vi "R ead.vi"(8 "error in (no error)":errorcluster, 10 "Start address":string, 11 "MelsecTCP in":refnum<class "MelsecMcNet.lvclass">) -> (0 "error out":errorcluster, 2 "Bools":bool, 3 "MelsecTCP out":refnum<class "MelsecMcNet.lvclass">)   [LabVIEW 2020]
uses:
  C:/Users/Fred Guo/Desktop/API_Salcomp_CMES/Libraries/HslCommunication/HslCommunication.dll
  HslCommunication.dll
  MelsecMcNet.lvclass
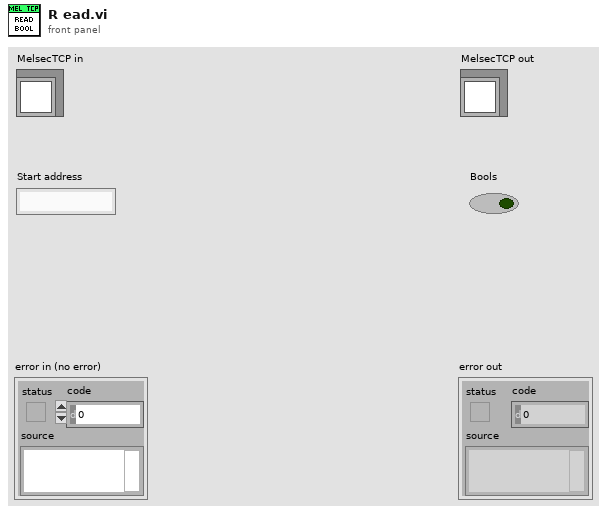
[diagram p1: front panel]
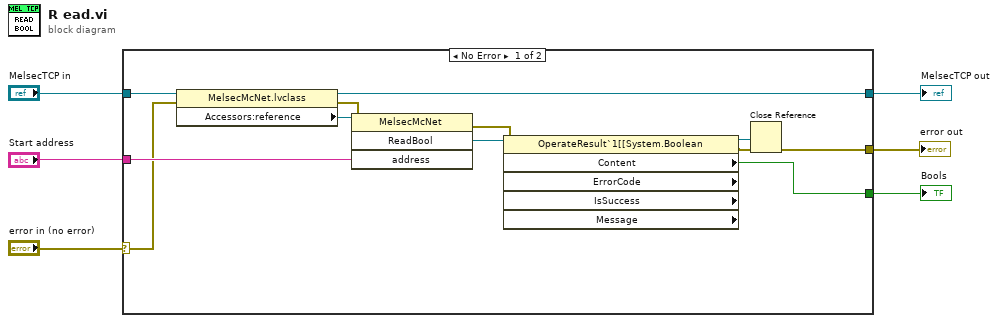
[diagram p0: block diagram]
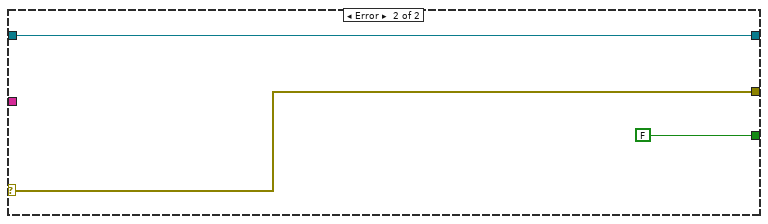
[diagram p2: hidden frame]
diagram:
  n1 = case shown="No Error" "error in (no error)" {
    selector: "error in (no error)" -> [w7 w21]
    tunnel: "MelsecTCP in" -> [w18 w19]
    tunnel: [w17 w19] -> w5
    tunnel: "Start address" -> [w15 _]
    tunnel: [w10 w21] -> w3
    tunnel: [w8 FALSE ("Content")] -> w2
    frame No Error {
      n2 = property class="MelsecMcNet.lvclass"(reference=w18, error in=w7) -> (reference out=w17:refnum<class "MelsecMcNet.lvclass">, error out=w13:errorcluster, "Accessors:reference"=w16:refnum<k24>)
      n3 = invoke class="MelsecMcNet" method="ReadBool"(reference=w16, error in=w13, "address"=w15) -> (error out=w12:errorcluster, "ReadBool"=w14:refnum<k24>)  [unwired: 1 in, 2 out]
      n4 = property class="OperateResult`1[[System.Boolean" props=["Content", "ErrorCode", "IsSuccess", "Message"](reference=w14, error in=w12) -> (reference out=w9:refnum<k24>, error out=w11:errorcluster, "Content"=w8:bool)  [unwired: 3 out]
      n5 = Close Reference(reference=w9, error in (no error)=w11) -> (error out=w10:errorcluster)
    }
    frame Error {
    }
  }
  "error out" <- w3
  "MelsecTCP out" <- w5
  "Bools" <- w2
